vi "pattern_from_sever.vi"(1 "Pattern Definition":T1={"X pitch"=35.0, "rotation"=0.0, "Center H"=-3.0, "Center V"=-32.0, "# Spots H"=6, "# Spots V"=4, "Spot size"=30.0, "ref_spot _dark"=TRUE, "Exact Phase Formula"=TRUE, "phase_wrap_pos"=TRUE, "Set Focus (mm)"=32.0, "phase_max"=4.0, "phase_factor"=56, "Steer LW"=1, "Steer vmax"=60, "phase_wrap_neg"=TRUE, "steer_horiz"=TRUE, "steer_pad"=0, "steer_only"=FALSE, "Wavelength"=6.28e-07, "Y pitch"=20.0, "python"=FALSE, "test_pattern"=FALSE, "grid"=TRUE, "dark_all"=FALSE, "Xm_str"="21.72,  44.87,  68.20,  91.45, 114.72, 137.87, 160.97, 184.04", "Ym_str"="21.72,  44.87,  68.20,  91.45, 114.72, 137.87, 160.97, 184.04", "ref_spot"=0, "stretch"=FALSE} {"ref_spot" min=0 max=500 step=1 format="%#.0f"; "Y pitch" min=0.0 max=100.0 format="%.2g"; "Wavelength" min=0.0 max=500.0 format="%^#.3e"; "steer_pad" min=0 max=500 step=1 format="%#.0f"; "Steer LW" max=500; "phase_max" min=0.0 max=500.0 format="%#.3f"; "Set Focus (mm)" min=0.0 max=500.0 format="%#.3g"; "Spot size" min=1.0 format="%.2g"; "# Spots V" min=1 step=1; "# Spots H" min=1 step=1; "Center V" format="%.2f"; "Center H" format="%.2f"; "rotation" min=-90.0 max=90.0 format="%.2g"; "X pitch" min=0.0 max=100.0 format="%.2g"}) -> (0 "data out":u8[][](array[numeric]))   [LabVIEW 2011]
uses:
  Periodic Spot Pattern Parameters.ctl
panel:
  out "Intensity Graph":u8[][](graph)
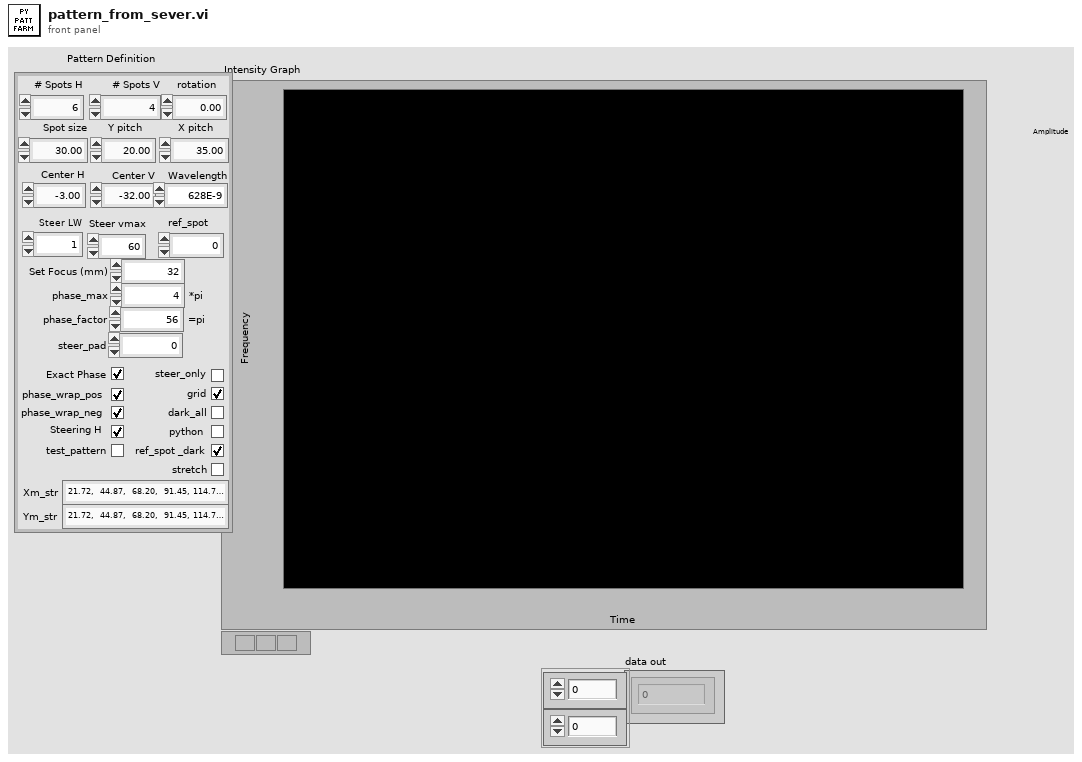
[diagram p1: front panel]
types:
  T1 = typedef "Periodic Spot Pattern Parameters.ctl" = cluster{"X pitch":dbl, "rotation":dbl, "Center H":dbl, "Center V":dbl, "# Spots H":u32, "# Spots V":u32, "Spot size":dbl, "ref_spot _dark":bool, "Exact Phase Formula":bool, "phase_wrap_pos":bool, "Set Focus (mm)":dbl, "phase_max":dbl, "phase_factor":u8, "Steer LW":u32, "Steer vmax":u8, "phase_wrap_neg":bool, "steer_horiz":bool, "steer_pad":i64, "steer_only":bool, "Wavelength":dbl, "Y pitch":dbl, "python":bool, "test_pattern":bool, "grid":bool, "dark_all":bool, "Xm_str":string, "Ym_str":string, "ref_spot":i64, "stretch":bool}
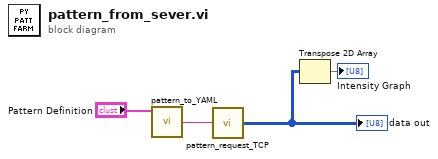
[diagram p0: block diagram]
diagram:
  n1 = call "pattern_to_YAML.vi"("Pattern Definition"="Pattern Definition") -> ("Result"=w4:string)  [unwired: 3 in]
  n2 = call "pattern_request_TCP.vi"("data in"=w4) -> ("data out"=w2:u8[][])
  "data out" <- w2
  n3 = Transpose 2D Array(2D array=w2) -> (transposed array=→"Intensity Graph":u8[][])
